vi "sendTriggersToWriteLoops.vi"(8 "error in":errorcluster, 9 "Trigger message":T2, 10 "Trigger queue enable array":bool[](array[boolean]), 11 "Trigger queue array":refnum<queue>[](array[refnum])) -> (0 "error out":errorcluster={"status"=TRUE, "code"=-8001, "source"=""})   [LabVIEW 2017]
doc: "Send a trigger signal to each queue in an arbitrary array of queues"
uses:
  Trigger message.ctl
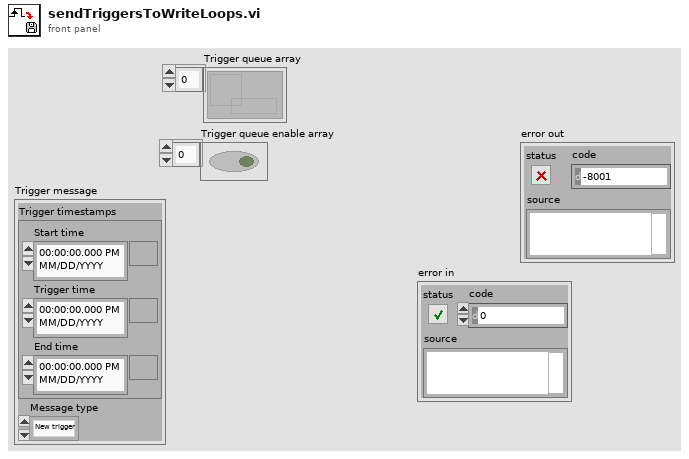
[diagram p1: front panel]
types:
  T1 = typedef "Trigger message.ctl" = enum16{"New trigger", "Updated trigger"}
  T2 = cluster{"Trigger timestamps":cluster{"Start time":timestamp, "Trigger time":timestamp, "End time":timestamp}, "Message type":T1}
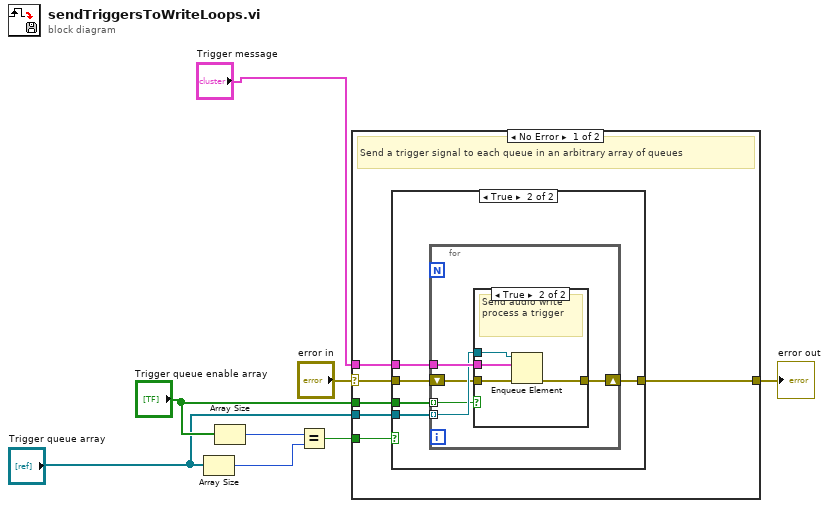
[diagram p0: block diagram]
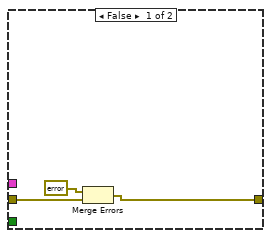
[diagram p2: hidden frame]
diagram:
  n1 = Array Size(array="Trigger queue array") -> (size(s)=w7:i32)
  n2 = Array Size(array="Trigger queue enable array") -> (size(s)=w6:i32)
  n3 = Equal?(x=w6, y=w7) -> (x = y?=w5:bool)
  n4 = case shown="No Error" "error in" {
    selector: "error in" -> [w9 w33]
    tunnel: "Trigger message" -> [w14 _]
    tunnel: "Trigger queue array" -> [w13 _]
    tunnel: "Trigger queue enable array" -> [w12 _]
    tunnel: w5 -> [w11 _]
    tunnel: [w10 w33] -> w4
    frame No Error {
      # "Send a trigger signal to each queue in an arbitrary array of queues"
      n5 = case shown="True" w11 {
        tunnel: w14 -> [_ w22]
        tunnel: w13 -> [_ w21]
        tunnel: w12 -> [_ w20]
        tunnel: [w15 w18] -> w10
        tunnel: w9 -> [w17 w19]
        frame False {
          n6 = Merge Errors(errorcluster {"status"=TRUE, "code"=-8001, "source"="Boolean and queue arrays must have the same sizew"} ("error constant"), w17) -> (w15:errorcluster)
        }
        frame True {
          n7 = for {
            tunnel: w22 -> [w27]
            tunnel: w21 -> [w26] mode=indexing
            tunnel: w20 -> [w25] mode=indexing
            shift-right: [w23] -> w18
            shift-left: w19 -> [w24]
            n8 = case shown="True" w25 {
              tunnel: w27 -> [_ w32]
              tunnel: w26 -> [_ w31]
              tunnel: w24 -> [w28 w30]
              tunnel: [w28 w29] -> w23
              frame False {
              }
              frame True {
                # "Send audio write \nprocess a trigger"
                n9 = Enqueue Element(queue=w31, element=w32, error in (no error)=w30) -> (error out=w29:errorcluster)  [unwired: 1 in, 2 out]
              }
            }
          }
        }
      }
    }
    frame Error {
    }
  }
  "error out" <- w4
